vi "SelScanFunc.vi"(4 "Function":i32, 6 "SInglePar":bool=TRUE, 8 "ErrorIn(No Error)":errorcluster caption="entrée d'erreur (pas d'erreur)", 9 "Active ScanPar":bool[](array[boolean]), 10 "ScanHeaderIn":i32[](array[numeric]), 11 "ScanIndexIn":i32[][](array[numeric])) -> (0 "sortie d'erreur":errorcluster, 2 "ScanHeaderOut":i32[](array[numeric]), 3 "ScanIndexOut":i32[][](array[numeric]))   [LabVIEW 2019]
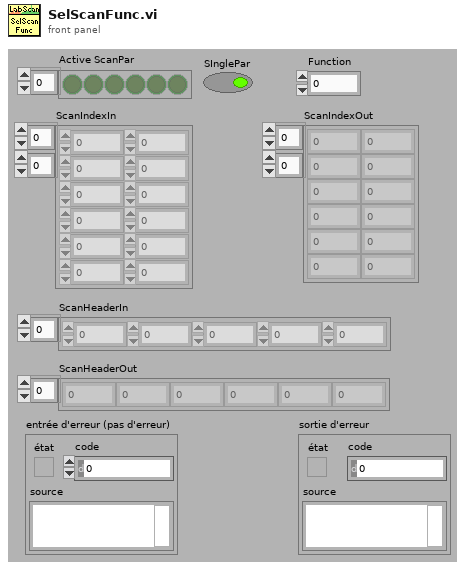
[diagram p1: front panel]
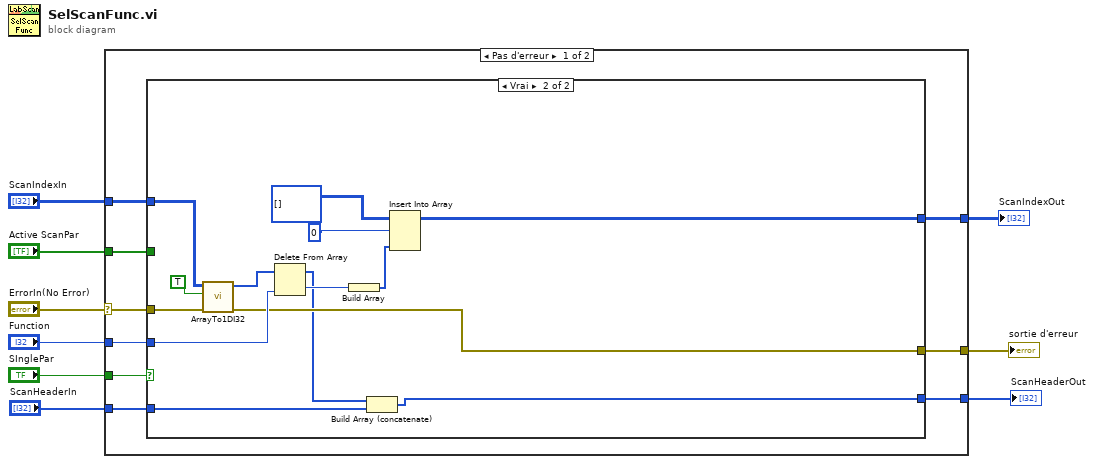
[diagram p0: block diagram]
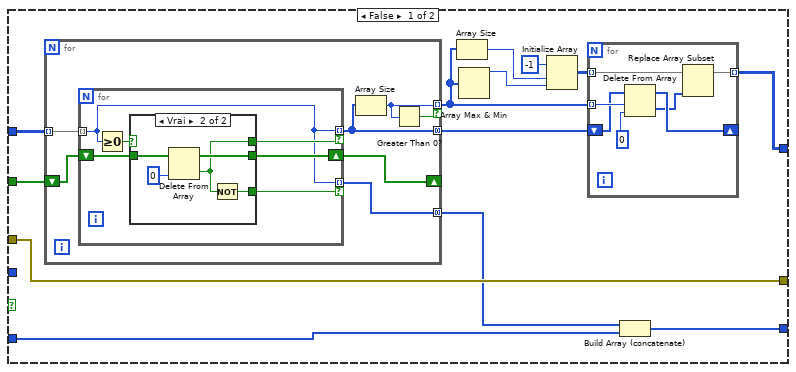
[diagram p2: hidden frame]
diagram:
  n1 = case shown="Pas d'erreur" "ErrorIn(No Error)" {
    selector: "ErrorIn(No Error)" -> [w13 w74]
    tunnel: [w12 w74] -> w8
    tunnel: "ScanIndexIn" -> [w15 _]
    tunnel: "Active ScanPar" -> [w14 _]
    tunnel: "SInglePar" -> [w17 _]
    tunnel: "Function" -> [w18 _]
    tunnel: [w16 _] -> w3
    tunnel: "ScanHeaderIn" -> [w11 w73]
    tunnel: [w10 w73] -> w1
    frame No Error {
      n2 = case shown="Vrai" w17 {
        tunnel: w15 -> [w31 w64]
        tunnel: w13 -> [w29 w70]
        tunnel: w18 -> [_ w69]
        tunnel: [w29 w62] -> w12
        tunnel: [w21 w63] -> w16
        tunnel: w14 -> [w30 _]
        tunnel: w11 -> [w28 w60]
        tunnel: [w26 w59] -> w10
        frame False {
          n3 = for {
            tunnel: w31 -> [w45] mode=indexing
            shift-right: [w43] -> _
            shift-left: w30 -> [w44]
            tunnel: [w42] -> w27 mode=concatenating
            tunnel: [w40] -> w20 mode=indexing if=w39
            tunnel: [w41] -> w25 mode=concatenating
            n4 = for {
              tunnel: w45 -> [w47] mode=indexing
              shift-right: [w50] -> w43
              shift-left: w44 -> [w51]
              tunnel: [w47] -> w41 mode=indexing if=w49
              tunnel: [w47] -> w42 mode=indexing if=w46
              n5 = Greater Or Equal To 0?(x=w47) -> (x >= 0?=w48:bool)
              n6 = case shown="Vrai" w48 {
                selector: w48 -> [w52 _]
                tunnel: w51 -> [w53 w58]
                tunnel: [w53 w56] -> w50
                tunnel: [w52 w55] -> w49
                tunnel: [w52 w54] -> w46
                frame False {
                  # "not in Active Arr"
                }
                frame True {
                  n7 = Delete From Array(array=w58, index=0 ("indice")) -> (deleted portion=w55:bool, array with subset deleted=w56:bool[])  [unwired: 1 in]
                  n8 = Not(x=w55) -> (.not. x?=w54:bool)
                }
              }
            }
            n9 = Array Size(array=w41) -> (size(s)=w40:i32)
            n10 = Greater Than 0?(x=w40) -> (x > 0?=w39:bool)
          }
          n11 = Array Size(array=w20) -> (size(s)=w19:i32)
          n12 = Array Max & Min(array=w20) -> (max value=w24:i32)  [unwired: 3 out]
          n13 = Initialize Array(-1, w19, w24) -> (w22:i32[][])
          n14 = for {
            tunnel: w20 -> [w38] mode=indexing
            tunnel: w22 -> [w35] mode=indexing
            shift-right: [w36] -> _
            shift-left: w25 -> [w37]
            tunnel: [w34] -> w21 mode=indexing
            n15 = Delete From Array(array=w37, length=w38, index=0 ("indice")) -> (deleted portion=w33:i32[], array with subset deleted=w36:i32[])
            n16 = Replace Array Subset(array=w35, new element=w33) -> (w34:i32[])  [unwired: 1 in]
          }
          n17 = Build Array (concatenate)(w27, w28) -> (w26:i32[])
        }
        frame True {
          n18 = call <userlib>:"ArrayTo1DI32.vi"("ErrorIn(No Error)"=w70, "DelArrEnd"=TRUE, "tableau"=w64) -> ("sortie d'erreur"=w62:errorcluster, "Array Out"=w72:i32[])  [unwired: 6 in, 1 out]
          n19 = Delete From Array(array=w72, index=w69) -> (deleted portion=w66:i32, array with subset deleted=w61:i32[])  [unwired: 1 in]
          n20 = Build Array(w66) -> (w65:i32[])
          n21 = Build Array (concatenate)(w61, w60) -> (w59:i32[])
          n22 = Insert Into Array(array=i32[][] [] ("ScanIndex"), index (row)=0 ("disabled index (col)"), new element=w65) -> (w63:i32[][])  [unwired: 1 in]
        }
      }
    }
    frame Error {
    }
  }
  "sortie d'erreur" <- w8
  "ScanIndexOut" <- w3
  "ScanHeaderOut" <- w1
